vi "AngleFinder.vi"(8 "wz":dbl, 9 "wy":dbl, 10 "wx":dbl, 11 "Array in":dbl[][](array[numeric])) -> (0 "Z":dbl, 1 "Y":dbl, 2 "X":dbl, 3 "Array out":dbl[][](array[numeric]))   [LabVIEW 2020]
uses:
  <vilib>/Analysis/NI_AALPro.lvlib
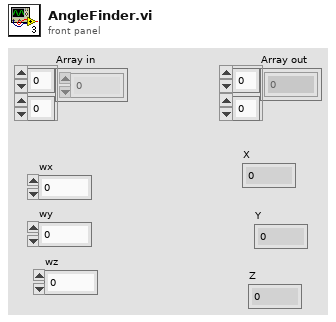
[diagram p1: front panel]
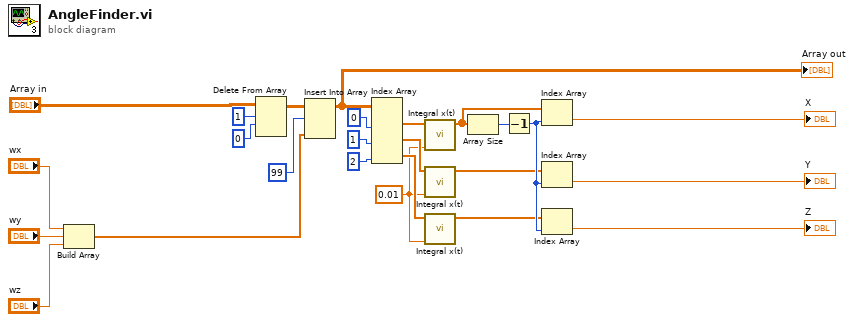
[diagram p0: block diagram]
diagram:
  w7 = 0.01 ("dt")
  n1 = Build Array("wx", "wy", "wz") -> (w23:dbl[])
  n2 = Delete From Array(array="Array in", length=1, index (row)=0) -> (array with subset deleted=w21:dbl[][])  [unwired: 1 in, 1 out]
  n3 = Insert Into Array(array=w21, index (row)=99, new element=w23) -> (w25:dbl[][])  [unwired: 1 in]
  "Array out" <- w25
  n4 = Index Array(array=w25, index (col) #1=0 ("disabled index (col)"), index (col) #2=1 ("index (col)"), index (col) #3=2 ("index (col)")) -> (element #1=w16:dbl[], element #2=w17:dbl[], element #3=w18:dbl[])  [unwired: 3 in]
  n5 = call <vilib>:"Integral x(t).vi"("dt"=w7, "X"=w16) -> ("Integral X"=w1:dbl[])  [unwired: 8 in, 1 out]
  n6 = call <vilib>:"Integral x(t).vi"("dt"=w7, "X"=w17) -> ("Integral X"=w3:dbl[])  [unwired: 8 in, 1 out]
  n7 = call <vilib>:"Integral x(t).vi"("dt"=w7, "X"=w18) -> ("Integral X"=w4:dbl[])  [unwired: 8 in, 1 out]
  n8 = Array Size(array=w1) -> (size(s)=w2:i32)
  n9 = Decrement(x=w2) -> (x-1=w8:i32)
  n10 = Index Array(array=w1, index=w8) -> (element=→"X":dbl)
  n11 = Index Array(array=w3, index=w8) -> (element=→"Y":dbl)
  n12 = Index Array(array=w4, index=w8) -> (element=→"Z":dbl)
